vi "Create From Basic Refs.vi"(8 "error in (no error)":errorcluster, 11 "CSM Basic Refs":T1) -> (0 "error out":errorcluster, 3 "CSM-Helper.lvclass":refnum<class "CSM-Helper.lvclass">)   [LabVIEW 2017, in "CSM-Helper.lvclass"]
doc: "### Create From Basic Refs.vi\n\n-- <b>Controls</b> --\n- <b>CSM Basic Refs</b>:\n\n-- <b>Indicators</b> --\n- <b>CSM-Helper.lvclass</b>:"
uses:
  CSM-Helper.lvclass
  Utility/CSM Basic Refs.ctl
  Utility/CSM Module Type.ctl
  CSM-Helper.lvclass/CSM-Helper.ctl
  Utility/CSM-Helper Utility.lvlib
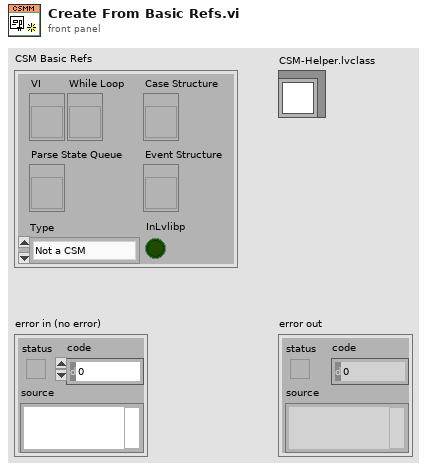
[diagram p1: front panel]
types:
  T1 = typedef "CSM-Helper Utility.lvlib/CSM Basic Refs.ctl" = cluster{"VI":refnum<vi>, "While Loop":refnum<vi>, "Case Structure":refnum<vi>, "Parse State Queue":refnum<vi>, "Event Structure":refnum<vi>, "Type":T2, "InLvlibp":bool}
  T2 = typedef "CSM-Helper Utility.lvlib/CSM Module Type.ctl" = enum16{"Not a CSM", "JKISM", "CSM"}
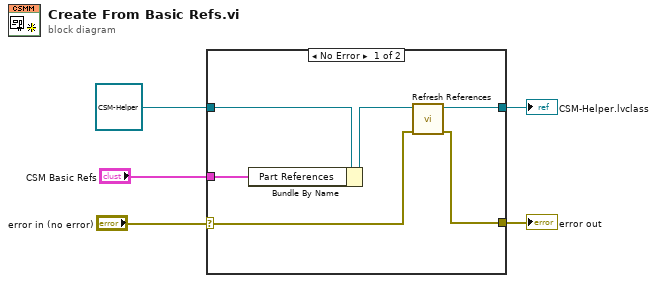
[diagram p0: block diagram]
diagram:
  n1 = case shown="No Error" "error in (no error)" {
    selector: "error in (no error)" -> [w6 w13]
    tunnel: [w9 w13] -> w4
    tunnel: [w10 w12] -> w2
    tunnel: refnum<class "CSM-Helper.lvclass"> refnum ("JKI SM") -> [w11 w12]
    tunnel: "CSM Basic Refs" -> [w7 _]
    frame No Error {
      n2 = Bundle By Name(cluster=w11, "Part References"=w7) -> (w8:refnum<class "CSM-Helper.lvclass">)
      n3 = call "Refresh References.vi"("error in (no error)"=w6, "CSM-Helper in"=w8) -> ("error out"=w9:errorcluster, "CSM-Helper out"=w10:refnum<class "CSM-Helper.lvclass">)  [unwired: 8 in]
    }
    frame Error {
    }
  }
  "error out" <- w4
  "CSM-Helper.lvclass" <- w2
